vi "Complex Cluster MsgPack Example.vi"() -> ()   [LabVIEW 2015, in "MsgPack.lvlib"]
uses:
  MsgPack.lvlib
  Complex Cluster.ctl
  Simple Cluster.ctl
panel:
  out "Top Key Found":bool
  in  "Top Level Key?":string="Version"
  in  "Nested Key?":string="Version"
  out "Nested Key Found":bool
  out "Received Packet":T1 {"ArrayOfClusters"."Single" format="%#.19f"; "NestedCluster"."Single" format="%#.19f"}
  out "Get Variant Attribute Error":errorcluster
  in  "Map to Cluster?(T)":bool=TRUE
  out "Decode Error":errorcluster
  out "Variant":variant
  in  "Cluster To Map? (T)":bool=TRUE
  in  "Flag":bool=TRUE
  in  "Compress? (T)":bool=TRUE
  out "MsgPack Data":string
  in  "Array Size":i32=20
  out "Packet":T1 {"ArrayOfClusters"."Single" format="%#.19f"; "NestedCluster"."Single" format="%#.19f"}
  # "This Example VI shows a way to send a complex Cluster over MsgPack.  This is an extenstion to the \"Simple Cluster MsgPack Example.vi\", Variant Attributes can be nested to form complex Clusters.\n\nFor this example to work without errors ensure the following parameters are TRUE:\n - Cluster To Map?\n - Map to Cluster?\n\n1 - The Time is autopopulated with the current timestamp.  This shows how the MsgPack EXT datatype can be used for sending custom data types.  A Timestamp (EXT type = -1) is defined by the MsgPack Standard and is included as an example.\n2 - Try setting different values for \"FLAG\" and \"Array Size\".\n3 - Toggle \"Compress?\"  to see the size difference in an array of integers\n4 - Toggle \"Cluster To Map?\" and \"Map To Cluster?\" to see how the MsgPack Data and resultant Variant are affected.\n5 - Try type in a new \"Key\" to see if it exists in the Variant on that particular level.\n\n\nNote: Use Get Variant Attributes with a Variant datatype to pull the \"nested Cluster\" and then simply use Get Variant Attributes to search for a specific Key on that level."
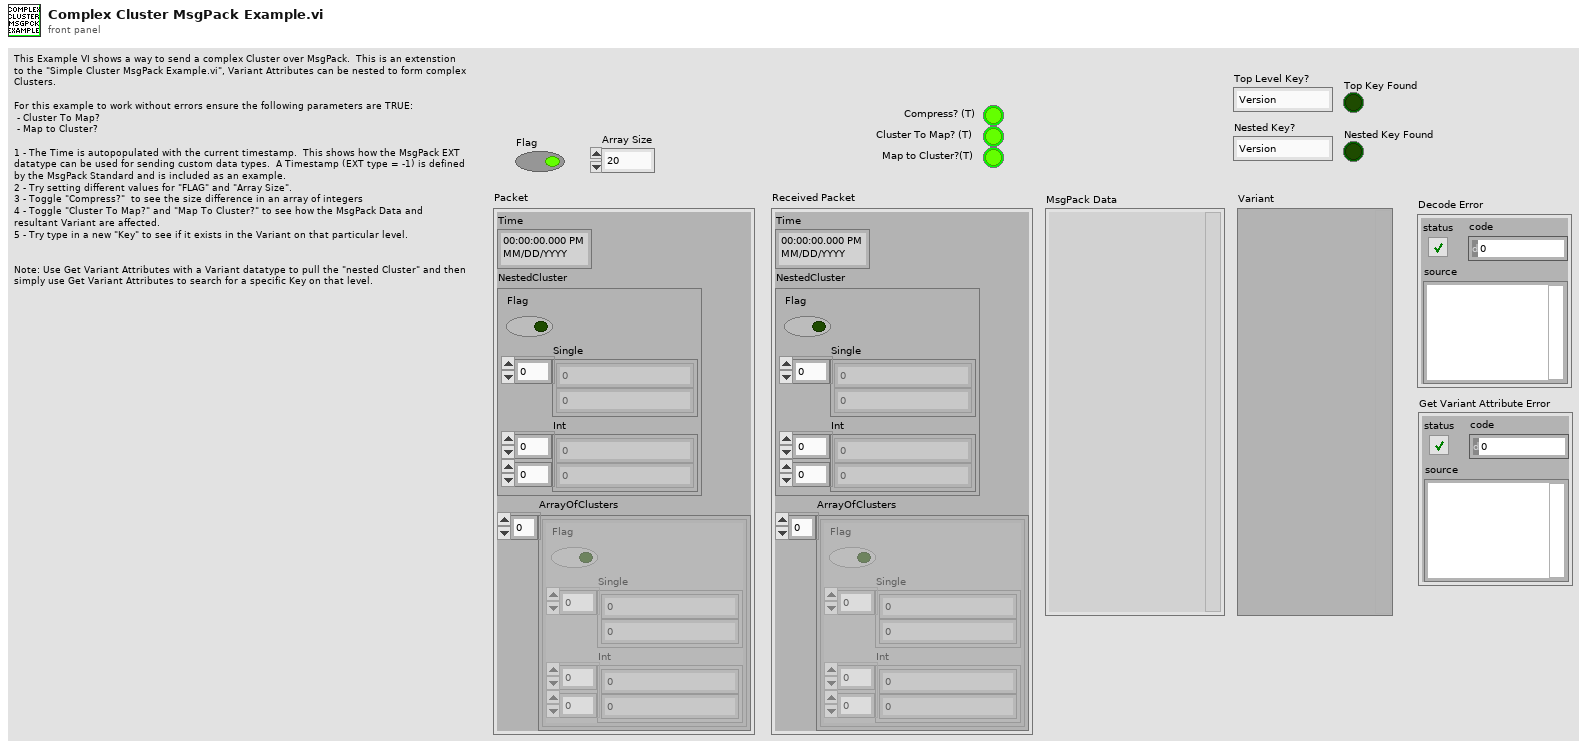
[diagram p1: front panel]
types:
  T1 = typedef "MsgPack.lvlib/Complex Cluster.ctl" = cluster{"Time":timestamp, "NestedCluster":T2, "ArrayOfClusters":T2[]}
  T2 = typedef "MsgPack.lvlib/Simple Cluster.ctl" = cluster{"Flag":bool, "Single":sgl[], "Int":i32[][]}
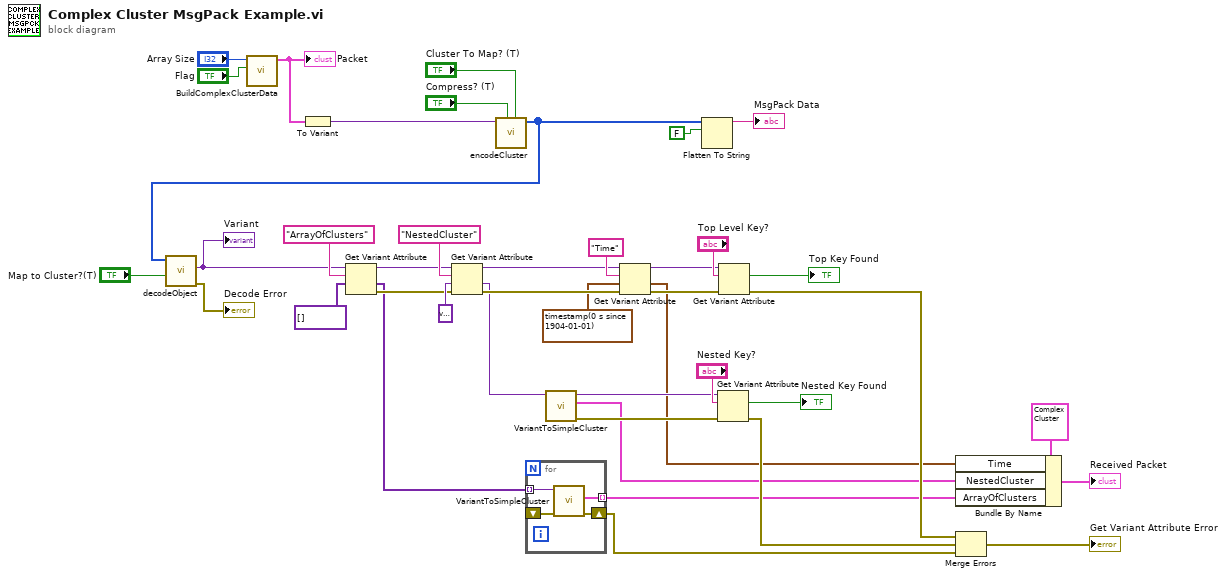
[diagram p0: block diagram]
diagram:
  n1 = call "BuildComplexClusterData.vi"("Flag"="Flag", "Array Size"="Array Size") -> ("Packet"=w1:T1)  [unwired: 9 in]
  "Packet" <- w1
  n2 = To Variant(anything=w1) -> (Variant=w38:variant)
  n3 = call "encodeCluster.vi"("Cluster To Map? [T]"="Cluster To Map? (T)", "Compress? (T)"="Compress? (T)", "Variant"=w38) -> ("MessagePack"=w33:u8[])  [unwired: 7 in, 1 out]
  n4 = call "decodeObject.vi"("Map to Cluster?(T)"="Map to Cluster?(T)", "ByteArray"=w33) -> ("error out"=→"Decode Error":errorcluster, "Variant"=w17:variant)  [unwired: 6 in, 2 out]
  "Variant" <- w17
  n5 = Get Variant Attribute(Variant=w17, name="ArrayOfClusters", default value (empty Variant)=variant[] []) -> (duplicate Variant=w18:variant, value=w13:variant[], error out=w16:errorcluster)  [unwired: 1 in, 1 out]
  n6 = Get Variant Attribute(Variant=w18, name="NestedCluster", default value (empty Variant)=variant, error in=w16) -> (duplicate Variant=w26:variant, value=w15:variant, error out=w27:errorcluster)  [unwired: 1 out]
  n7 = for {
    tunnel: w13 -> [w43] mode=indexing
    shift-right: [w45] -> w7
    shift-left: _ -> [w44]
    tunnel: [w42] -> w2 mode=indexing
    n8 = call "VariantToSimpleCluster.vi"("error in (no error)"=w44, "Variant"=w43) -> ("error out"=w45:errorcluster, "SimpleCluster"=w42:T2)  [unwired: 7 in, 1 out]
  }
  n9 = call "VariantToSimpleCluster.vi"("Variant"=w15) -> ("error out"=w11:errorcluster, "SimpleCluster"=w3:T2, "Variant (dup)"=w12:variant)  [unwired: 8 in]
  n10 = Get Variant Attribute(Variant=w26, name="Time", default value (empty Variant)=timestamp(0 s since 1904-01-01), error in=w27) -> (duplicate Variant=w23:variant, value=w5:timestamp, error out=w22:errorcluster)  [unwired: 1 out]
  n11 = Flatten To String(anything=w33, prepend array or string size? (T)=FALSE) -> (data string=→"MsgPack Data":string)  [unwired: 2 in, 2 out]
  n12 = Get Variant Attribute(Variant=w12, name="Nested Key?", error in=w11) -> (found=→"Nested Key Found":bool, error out=w8:errorcluster)  [unwired: 1 in, 2 out]
  n13 = Get Variant Attribute(Variant=w23, name="Top Level Key?", error in=w22) -> (found=→"Top Key Found":bool, error out=w9:errorcluster)  [unwired: 1 in, 2 out]
  n14 = Bundle By Name(cluster=T1 {"Time"=timestamp(0 s since 1904-01-01), "NestedCluster"={"Flag"=FALSE, "Single"=[], "Int"=[]}, "ArrayOfClusters"=[]} ("Packet"), "Time"=w5, "NestedCluster"=w3, "ArrayOfClusters"=w2) -> (→"Received Packet":T1)
  n15 = Merge Errors(w9, w8, w7) -> (→"Get Variant Attribute Error":errorcluster)
